vi "Connect.vi"(8 "error in (no error)":errorcluster, 10 "Password":string, 11 "SSID":string) -> (0 "error out":errorcluster, 3 "Feedback":string)   [LabVIEW 2012]
doc: "Connects to a wireless network by using the specified parameter."
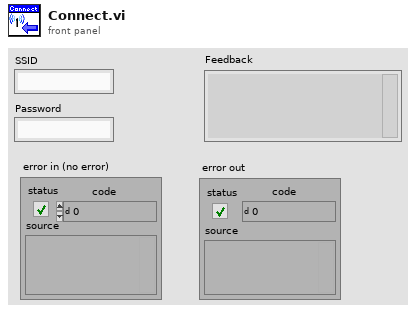
[diagram p1: front panel]
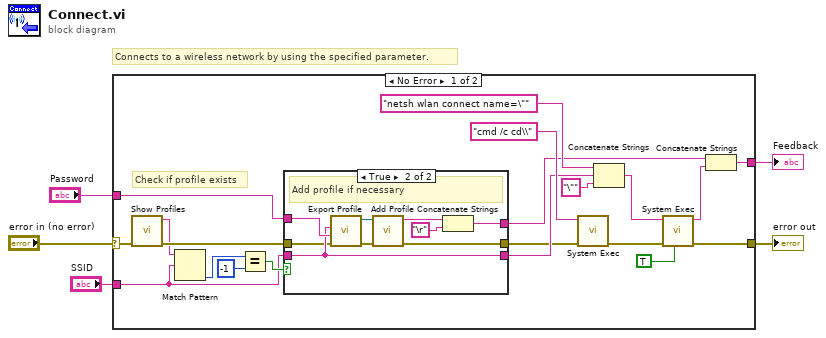
[diagram p0: block diagram]
diagram:
  # "Connects to a wireless network by using the specified parameter."
  n1 = case shown="No Error" "error in (no error)" {
    selector: "error in (no error)" -> [w6 w37]
    tunnel: [w12 w37] -> w5
    tunnel: [w11 _] -> w4
    tunnel: "SSID" -> [w22 _]
    tunnel: "Password" -> [w21 _]
    frame No Error {
      # "Check if profile exists"
      n2 = call "Show Profiles.vi"("error in (no error)"=w6) -> ("error out"=w8:errorcluster, "Feedback"=w7:string)  [unwired: 9 in]
      n3 = Match Pattern(string=w7, regular expression=w22) -> (offset past match=w25:i32)  [unwired: 1 in, 3 out]
      n4 = Equal?(x=w25, y=-1) -> (x = y?=w23:bool)
      n5 = case shown="True" w23 {
        tunnel: w22 -> [w27 w33]
        tunnel: [w26 w32] -> w13
        tunnel: w8 -> [w26 w28]
        tunnel: [w27 w33] -> w14
        tunnel: w21 -> [_ w34]
        tunnel: [_ w35] -> w10
        frame False {
          # "Profile already existing"
        }
        frame True {
          # "Add profile if necessary"
          n6 = call "Export Profile.vi"("error in (no error)"=w28, "Password"=w34, "SSID"=w33) -> ("error out"=w31:errorcluster, "XML path out"=w30:path)  [unwired: 6 in, 1 out]
          n7 = call "Add Profile.vi"("error in (no error)"=w31, "Path"=w30) -> ("error out"=w32:errorcluster, "Feedback"=w29:string)  [unwired: 8 in]
          n8 = Concatenate Strings(w29, "\r") -> (w35:string)
        }
      }
      n9 = call <vilib>:"System Exec.vi"("error in (no error)"=w13, "command line"="cmd /c cd\\") -> ("error out"=w20:errorcluster)  [unwired: 6 in, 3 out]
      n10 = Concatenate Strings("netsh wlan connect name=\"" ("command line"), w14, "\"" ("string")) -> (w19:string)
      n11 = call <vilib>:"System Exec.vi"("run minimized? (F)"=TRUE, "error in (no error)"=w20, "command line"=w19) -> ("error out"=w12:errorcluster, "standard output"=w9:string)  [unwired: 5 in, 2 out]
      n12 = Concatenate Strings(w10, w9) -> (w11:string)
    }
    frame Error {
    }
  }
  "error out" <- w5
  "Feedback" <- w4
